vi "Test sub panel.vi"() -> ()   [LabVIEW 2015]
uses:
  Instruments/LakeShore/LakeShore370/LakeShore370_device.lvclass
  Device/Device.lvclass
panel:
  in  "stop":bool
  in  "Numeric":dbl
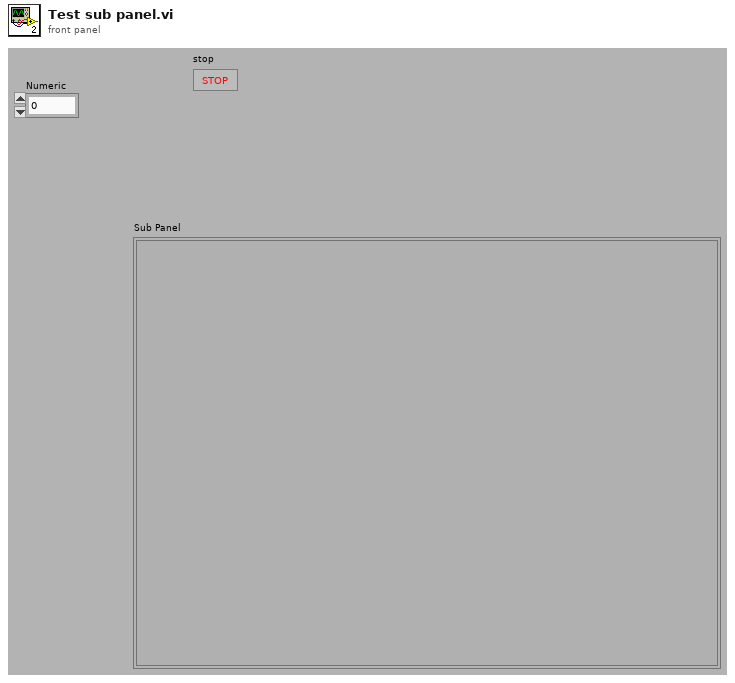
[diagram p1: front panel]
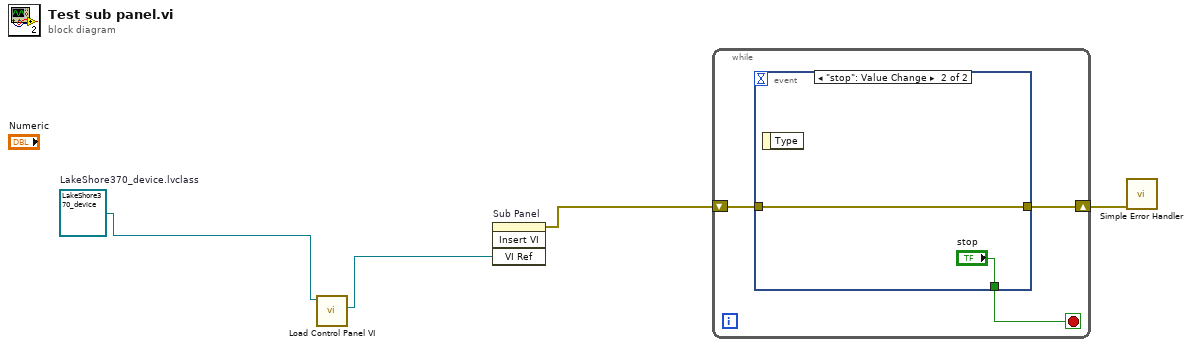
[diagram p0: block diagram]
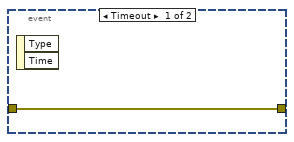
[diagram p2: hidden frame]
diagram:
  w1 = refnum<class "LakeShore370_device.lvclass"> refnum  # LakeShore370_device.lvclass
  n1 = call "Load Control Panel VI.vi"("Device"=w1) -> ("vi ref out"=w4:refnum<vi>)  [unwired: 8 in, 2 out]
  n2 = invoke on="Sub Panel" class="SubPanel" method="Insert VI"("VI Ref"=w4) -> (error out=w3:errorcluster)  [unwired: 3 in, 3 out]
  n3 = while {
    shift-right: [w6] -> w2
    shift-left: w3 -> [w7]
    stop <- w5 stop-if-true
    n4 = event shown="[1] \"stop\": Value Change" {
      selector: _ -> [_ _]
      dyn-events: _ -> [_ _]
      timeout: _ -> [_ _]
      tunnel: w7 -> [w8 w10]
      tunnel: [w8 w10] -> w6
      tunnel: [_ "stop"] -> w5
      event Timeout {
        n5 = event-data() -> ()  [unwired: 1 in, 2 out]
      }
      event "stop": Value Change {
        n6 = event-data() -> ()  [unwired: 1 in, 1 out]
      }
    }
  }
  n7 = call <vilib>:"Simple Error Handler.vi"("error in (no error)"=w2) -> ()  [unwired: 4 in, 5 out]
